vi "New.vi"(8 "error in (no error)":errorcluster, 10 "Options":string="{}", 11 "Procedure URI":string) -> (0 "error out":errorcluster, 2 "Result notifier":refnum<notifier>, 3 "Register JSON out":refnum<class "Register JSON.lvclass">)   [LabVIEW 2020, in "wamplv.lvlib" / "Register JSON.lvclass"]
uses:
  Register JSON.lvclass
  WAMP Client/API/TypeDefs/Error or abort detail (JSON).ctl
  wamplv.lvlib
  WAMP Client/Private/TypeDef/Success or error (JSON).ctl
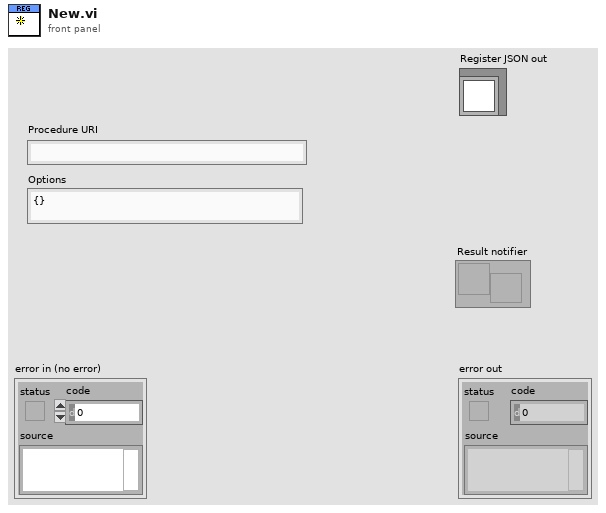
[diagram p1: front panel]
types:
  T1 = typedef "wamplv.lvlib/Success or error (JSON).ctl" = cluster{"Success?":bool, "URI":string, "Error/Abort details (JSON)":T2}
  T2 = typedef "wamplv.lvlib/Error or abort detail (JSON).ctl" = cluster{"Error URI":string, "Error Arguments":string, "Error ArgumentKw":string, "Error Details":string}
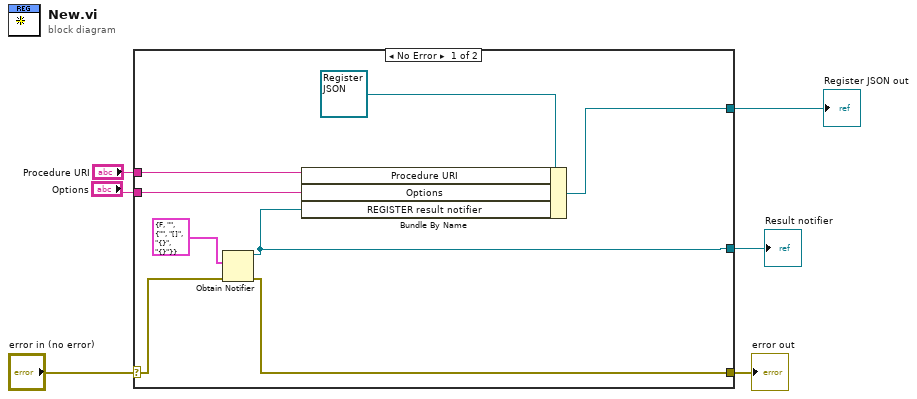
[diagram p0: block diagram]
diagram:
  n1 = case shown="No Error" "error in (no error)" {
    selector: "error in (no error)" -> [w12 w15]
    tunnel: [w11 w15] -> w5
    tunnel: "Procedure URI" -> [w14 _]
    tunnel: "Options" -> [w13 _]
    tunnel: [w8 _] -> w2
    tunnel: [w9 _] -> w1
    frame No Error {
      n2 = Obtain Notifier(notification data type=T1 {"Success?"=FALSE, "URI"="", "Error/Abort details (JSON)"={"Error URI"="", "Error Arguments"="[]", "Error ArgumentKw"="{}", "Error Details"="{}"}} ("Sucess or error (JSON)"), error in (no error)=w12) -> (notifier out=w8:refnum<notifier>, error out=w11:errorcluster)  [unwired: 2 in, 1 out]
      n3 = Bundle By Name(cluster=refnum<class "Register JSON.lvclass"> refnum ("wamplv.lvlib:Register JSON.lvclass"), "Procedure URI"=w14, "Options"=w13, "REGISTER result notifier"=w8) -> (w9:refnum<class "Register JSON.lvclass">)
    }
    frame Error {
    }
  }
  "error out" <- w5
  "Register JSON out" <- w1
  "Result notifier" <- w2
